vi "EST.Output.Generate.vi"(8 "error in (no error)":errorcluster, 11 "Parameters":T2) -> (0 "error out":errorcluster, 3 "Output.Ref":refnum<vi>)   [LabVIEW 2015]
uses:
  <vilib>/Utility/miscctls.llb/LVPointTypeDef.ctl
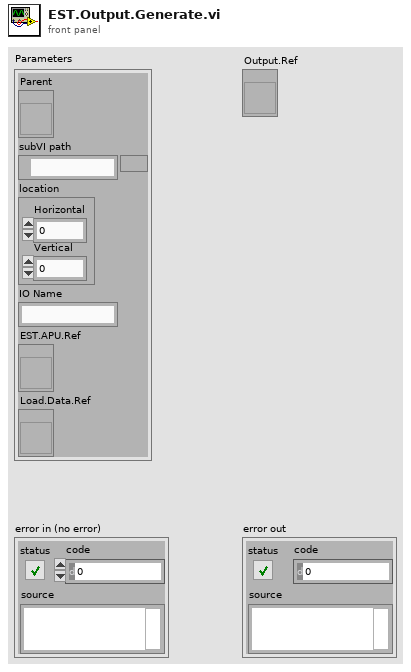
[diagram p1: front panel]
types:
  T1 = typedef "LVPointTypeDef.ctl" = cluster{"Horizontal":i16, "Vertical":i16}
  T2 = cluster{"Parent":refnum<vi>, "subVI path":path, "location":T1, "IO Name":string, "EST.APU.Ref":refnum<vi>, "Load.Data.Ref":refnum<vi>}
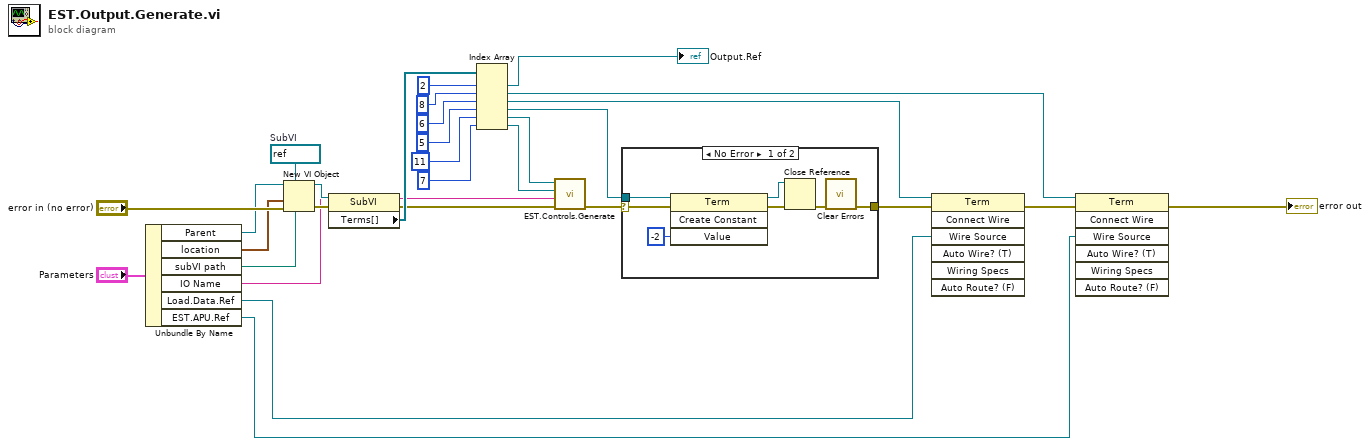
[diagram p0: block diagram]
diagram:
  w23 = refnum<vi> refnum  # SubVI
  n1 = Unbundle By Name("Parameters") -> ("Parent"=w21:refnum<vi>, "location"=w20:T1, "subVI path"=w19:path, "IO Name"=w5:string, "Load.Data.Ref"=w6:refnum<vi>, "EST.APU.Ref"=w7:refnum<vi>)
  n2 = New VI Object(vi object class=w23, owner refnum=w21, position/next to=w20, 6:w19, 8:"error in (no error)") -> (object refnum=w27:refnum<vi>, 0:w28:errorcluster)  [unwired: 3 in]
  n3 = property class="SubVI"(reference=w27, error in=w28) -> (error out=w2:errorcluster, "Terms[]"=w25:refnum<vi>[])  [unwired: 1 out]
  n4 = Index Array(array=w25, index #1=2 ("index"), index #2=8 ("index"), index #3=6 ("index"), index #4=5 ("index"), index #5=11 ("index"), index #6=7 ("index")) -> (element #1=→"Output.Ref":refnum<vi>, element #2=w8:refnum<vi>, element #3=w13:refnum<vi>, element #4=w15:refnum<vi>, element #5=w3:refnum<vi>, element #6=w4:refnum<vi>)
  n5 = call "EST.Controls.Generate.vi"("error in (no error)"=w2, "IO Name"=w5, "Input.Ref"=w4, "Settings.Ref"=w3) -> ("error out"=w1:errorcluster)  [unwired: 7 in]
  n6 = case shown="No Error" w1 {
    selector: w1 -> [w34 w37]
    tunnel: w15 -> [w36 _]
    tunnel: [w30 w37] -> w14
    frame No Error {
      n7 = invoke class="Term" method="Create Constant"(reference=w36, error in=w34, "Value"=i8 -2 ("shift")) -> (reference out=w32:refnum<vi>, error out=w33:errorcluster)  [unwired: 1 in, 2 out]
      n8 = Close Reference(reference=w32, error in (no error)=w33) -> (error out=w31:errorcluster)
      n9 = call <vilib>:"Clear Errors.vi"("error in (no error)"=w31) -> ("error out"=w30:errorcluster)  [unwired: 5 in, 1 out]
    }
    frame Error {
    }
  }
  n10 = invoke class="Term" method="Connect Wire"(reference=w13, error in=w14, "Wire Source"=w6) -> (error out=w10:errorcluster)  [unwired: 4 in, 6 out]
  n11 = invoke class="Term" method="Connect Wire"(reference=w8, error in=w10, "Wire Source"=w7) -> (error out=→"error out":errorcluster)  [unwired: 4 in, 6 out]
